vi "MeasureQueue.vi"() -> ()   [LabVIEW 2017]
uses:
  MeasureQueue.ctl
  MeasureMessage.ctl
panel:
  in  "MeasureQueue":T1
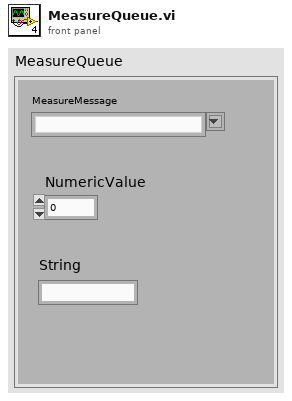
[diagram p1: front panel]
types:
  T1 = typedef "MeasureQueue.ctl" = cluster{"MeasureMessage":T2, "NumericValue":dbl, "String":string}
  T2 = typedef "MeasureMessage.ctl" = string
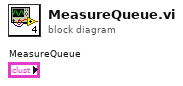
[diagram p0: block diagram]
diagram:
